vi "DAQmx Read (Digital U8 1Chan 1Samp).vi"(0 "task/channels in":refnum<k21>, 9 "timeout":dbl=10.0 format="%0.2f", 11 "error in":errorcluster) -> (4 "task out":refnum<k21>, 6 "data":u8, 15 "error out":errorcluster)   [LabVIEW 2017]
doc: "Reads a single 8-bit unsigned integer sample from a task that contains a single digital input channel. Use an instance that reads 8-bit unsigned integers for devices with up to eight lines per port."
uses:
  nilvaiu.dll
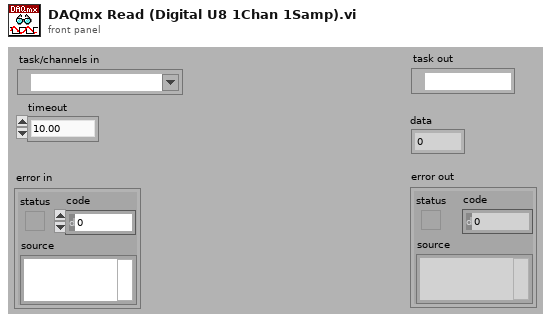
[diagram p1: front panel]
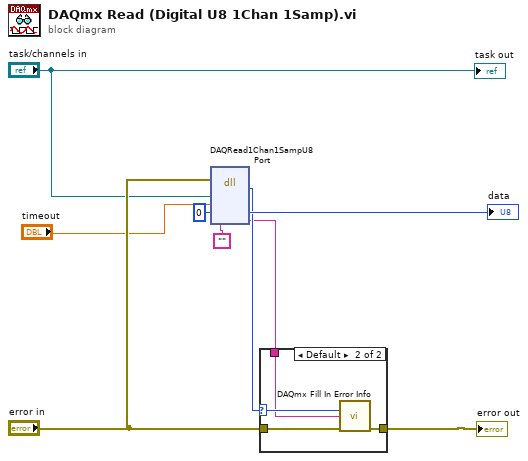
[diagram p0: block diagram]
diagram:
  n1 = dll-call lib="nilvaiu.*" fn="DAQRead1Chan1SampU8Port"(error in="error in", "taskID"="task/channels in", "timeout"="timeout", "data"=u8 0, "extendedErrorInfo"="") -> (w4:i32, "data"=→"data":u8, "extendedErrorInfo"=w2:string)  [unwired: 3 in, 3 out]
  n2 = case shown="Default" w4 {
    selector: w4 -> [_ w12]
    tunnel: "error in" -> [w10 w14]
    tunnel: [w10 w13] -> w8
    tunnel: w2 -> [_ w11]
    frame 0 {
    }
    frame Default {
      n3 = call "DAQmx Fill In Error Info.vi"("status code"=w12, "extended error info"=w11, "error in"=w14) -> ("error out"=w13:errorcluster)  [unwired: 1 in, 11 out]
    }
  }
  "error out" <- w8
  "task out" <- "task/channels in"
